vi "clearEventLog.vi"(8 "error in (no error)":errorcluster, 11 "Text reference":refnum<vi>) -> (0 "error out":errorcluster)   [LabVIEW 2017]
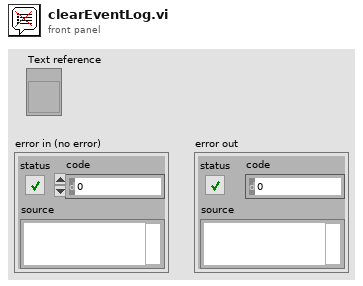
[diagram p1: front panel]
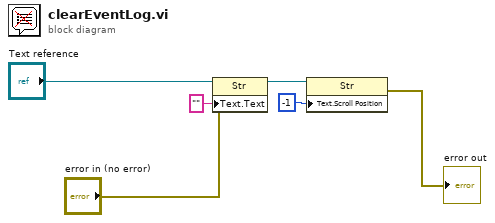
[diagram p0: block diagram]
diagram:
  n1 = property class="Str"(reference="Text reference", error in="error in (no error)", "Text.Text"="") -> (reference out=w5:refnum<vi>)  [unwired: 1 out]
  n2 = property class="Str"(reference=w5, "Text.Scroll Position"=-1) -> (error out=→"error out":errorcluster)  [unwired: 1 in, 1 out]
